vi "Create Batch Request.vi"(8 "error in (no error)":errorcluster, 10 "Requests":T1[](array[typedef]), 11 "JSON-RPC in":refnum<class "JSON-RPC.lvclass">) -> (0 "error out":errorcluster, 2 "Request":string, 3 "JSON-RPC out":refnum<class "JSON-RPC.lvclass">)   [LabVIEW 2019, in "JSON-RPC.lvclass"]
uses:
  JSON-RPC.lvclass
  typedefs/Request--Cluster.ctl
  JSON-RPC.lvclass/JSON-RPC.ctl
  Request/Request.lvclass
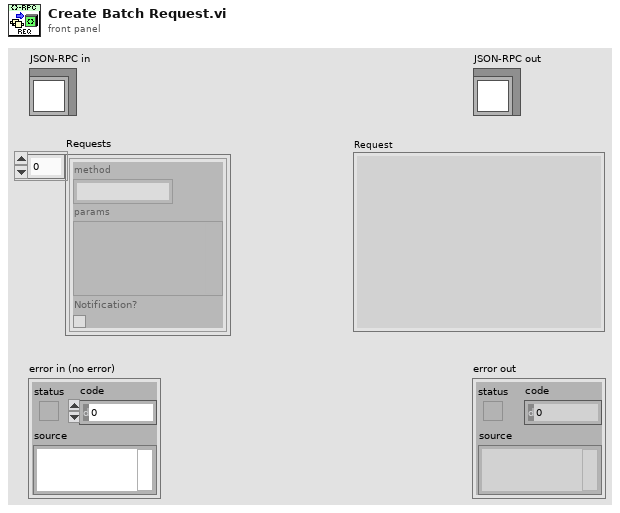
[diagram p1: front panel]
types:
  T1 = typedef "JSON-RPC.lvclass/Request--Cluster.ctl" = cluster{"method":string, "params":variant, "Notification?":bool}
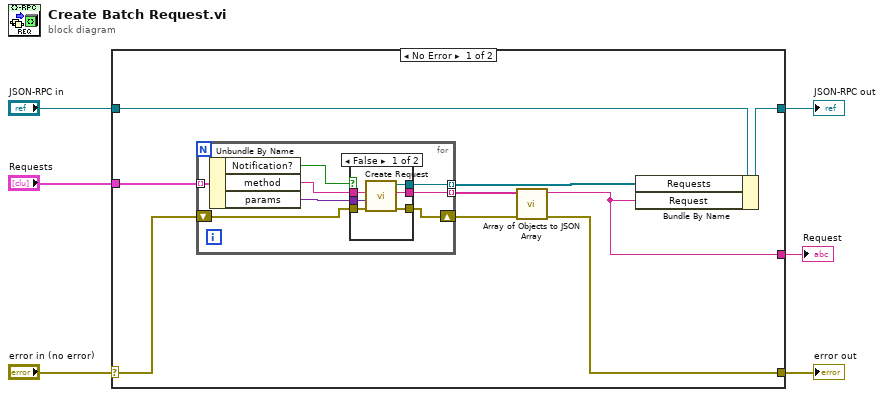
[diagram p0: block diagram]
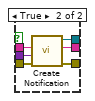
[diagram p2: hidden frame]
diagram:
  n1 = case shown="No Error" "error in (no error)" {
    selector: "error in (no error)" -> [w12 w37]
    tunnel: [w8 w37] -> w5
    tunnel: [w13 w36] -> w3
    tunnel: "JSON-RPC in" -> [w14 w36]
    tunnel: [w7 _] -> w2
    tunnel: "Requests" -> [w11 _]
    frame No Error {
      n2 = for {
        tunnel: [w23] -> w15 mode=indexing
        shift-right: [w21] -> w9
        shift-left: w12 -> [w22]
        tunnel: [w20] -> w10 mode=indexing
        tunnel: w11 -> [w19] mode=indexing
        n3 = Unbundle By Name(w19) -> ("Notification?"=w18:bool, "method"=w17:string, "params"=w16:variant)
        n4 = case shown="False" w18 {
          tunnel: [w29 w31] -> w23
          tunnel: w17 -> [w28 w33]
          tunnel: w16 -> [w27 w34]
          tunnel: w22 -> [w26 w35]
          tunnel: [w25 w30] -> w21
          tunnel: [w24 w32] -> w20
          frame False {
            n5 = call "Create Request.vi"("error in (no error)"=w26, "params"=w27, "method"=w28) -> ("error out"=w25:errorcluster, "JSON Request"=w24:string, "Request out"=w29:refnum<class "Request.lvclass">)  [unwired: 6 in]
          }
          frame True {
            n6 = call "Create Notification.vi"("error in (no error)"=w35, "params"=w34, "method"=w33) -> ("error out"=w30:errorcluster, "JSON Notificaiton"=w32:string, "Request"=w31:refnum<class "Request.lvclass">)  [unwired: 6 in]
          }
        }
      }
      n7 = call "Array of Objects to JSON Array.vi"("error in (no error)"=w9, "Array of JSON"=w10) -> ("error out"=w8:errorcluster, "JSON Array"=w7:string)  [unwired: 8 in]
      n8 = Bundle By Name(cluster=w14, "Requests"=w15, "Request"=w7) -> (w13:refnum<class "JSON-RPC.lvclass">)
    }
    frame Error {
    }
  }
  "error out" <- w5
  "JSON-RPC out" <- w3
  "Request" <- w2
